vi "Q_daq-data.vi"(7 "cmd":enum16{"create", "wirte", "read", "close"}(ring), 8 "error in":errorcluster, 11 "Q_data":T1) -> (0 "error out":errorcluster caption="erro out", 3 "queue out":refnum<queue>)   [LabVIEW 2013]
uses:
  ctl/q_data.ctl
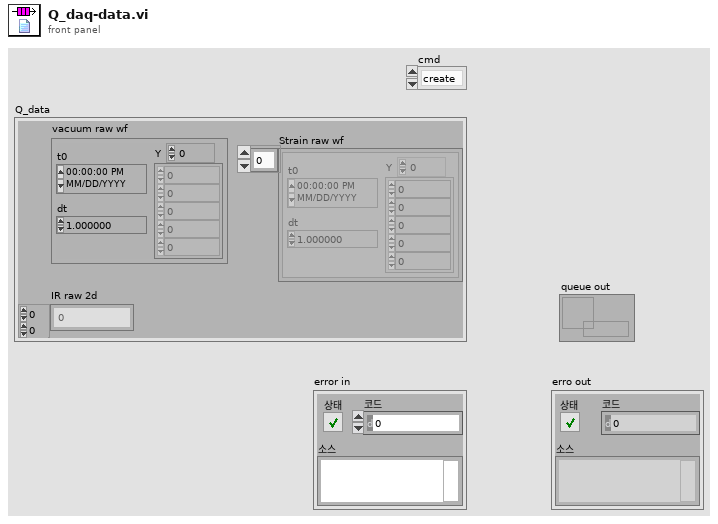
[diagram p1: front panel]
types:
  T1 = typedef "q_data.ctl" = cluster{"Strain raw wf":waveform(dbl)[], "vacuum raw wf":waveform(dbl), "IR raw 2d":i16[][]}
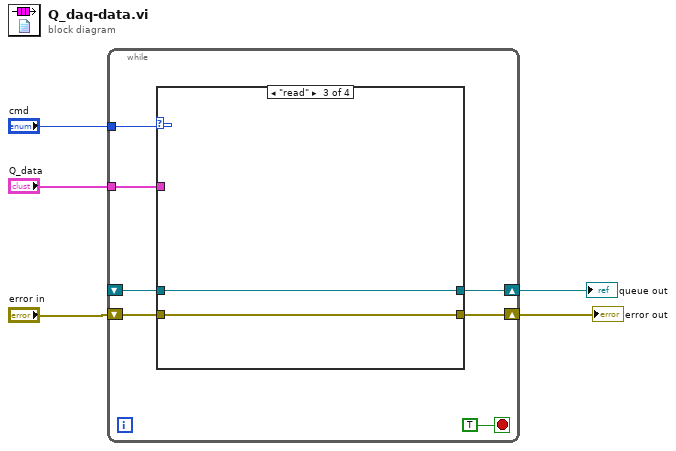
[diagram p0: block diagram]
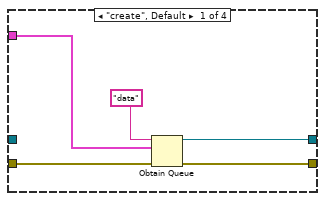
[diagram p2: hidden frame]
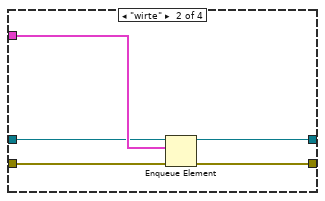
[diagram p3: hidden frame]
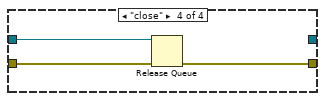
[diagram p4: hidden frame]
diagram:
  n1 = while {
    tunnel: "cmd" -> [w11]
    shift-right: [w9] -> w3
    shift-left: "error in" -> [w10]
    tunnel: "Q_data" -> [w8]
    shift-right: [w7] -> w1
    shift-left: _ -> [w6]
    stop <- TRUE stop-if-true
    n2 = case shown="\"read\"" w11 {
      tunnel: w10 -> [w16 w21 w24 w27]
      tunnel: [w15 w20 w24 w26] -> w9
      tunnel: w8 -> [w14 w22 _ _]
      tunnel: [w13 w19 w23 _] -> w7
      tunnel: w6 -> [_ w18 w23 w25]
      frame "create", Default {
        n3 = Obtain Queue(name (unnamed)="data" ("이름(이름없음)"), element data type=w14, error in (no error)=w16) -> (queue out=w13:refnum<queue>, error out=w15:errorcluster)  [unwired: 2 in, 1 out]
      }
      frame "wirte" {
        n4 = Enqueue Element(queue=w18, element=w22, error in (no error)=w21) -> (queue out=w19:refnum<queue>, error out=w20:errorcluster)  [unwired: 1 in, 1 out]
      }
      frame "read" {
      }
      frame "close" {
        n5 = Release Queue(queue=w25, error in (no error)=w27) -> (error out=w26:errorcluster)  [unwired: 1 in, 2 out]
      }
    }
  }
  "error out" <- w3
  "queue out" <- w1
